vi "Set Controls Enable or Disable State Data Recorder.vi"(8 "error in (no error)":errorcluster, 10 "Refnum State":T2=enum."Start Live", 11 "Refnums In":T1) -> (0 "error out":errorcluster)   [LabVIEW 2017]
uses:
  Controls/Enabled State Control.ctl
  Controls/Refnums.ctl
  Controls/Recording Settings.ctl
  Controls/Operator Settings.ctl
  Controls/Operator.ctl
  Controls/Patient Settings.ctl
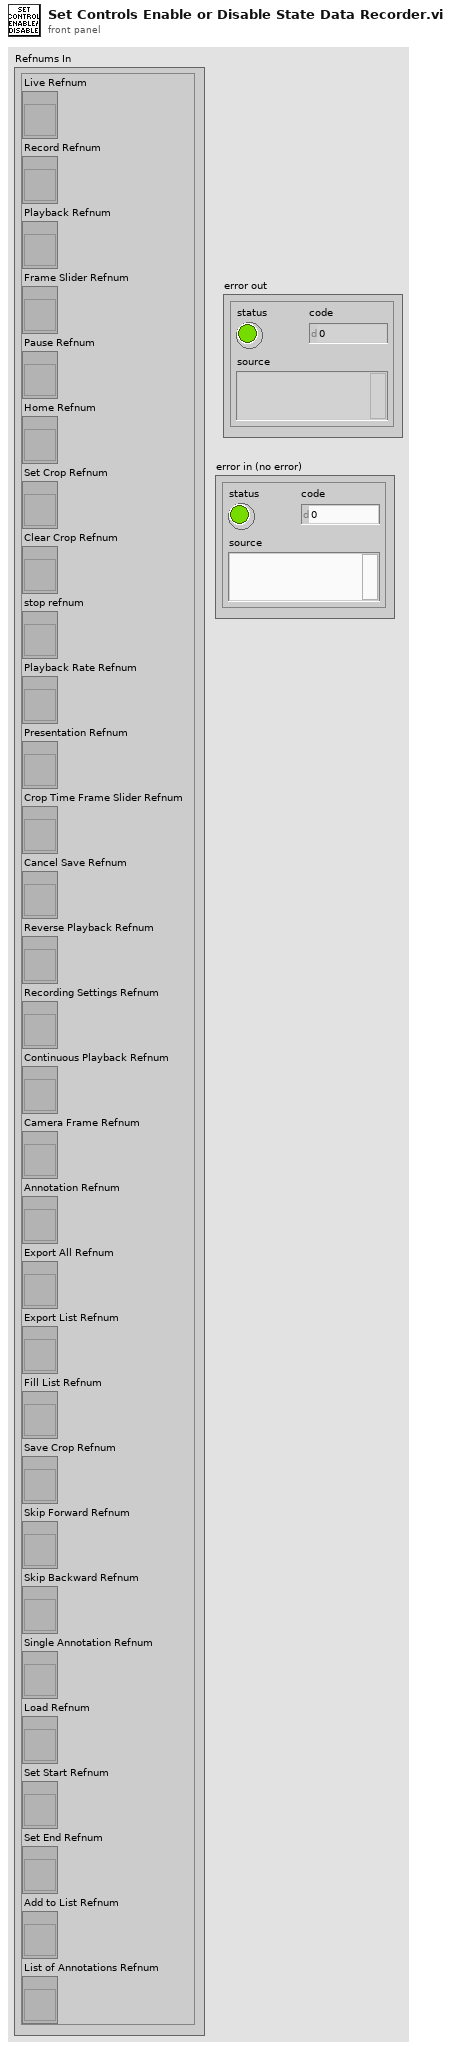
[diagram p1: front panel]
types:
  T1 = typedef "Refnums.ctl" = cluster{"Live Refnum":refnum<vi>, "Record Refnum":refnum<vi>, "Playback Refnum":refnum<vi>, "Frame Slider Refnum":refnum<vi>, "Pause Refnum":refnum<vi>, "Home Refnum":refnum<vi>, "Set Crop Refnum":refnum<vi>, "Clear Crop Refnum":refnum<vi>, "stop refnum":refnum<vi>, "Playback Rate Refnum":refnum<vi>, "Presentation Refnum":refnum<vi>, "Crop Time Frame Slider Refnum":refnum<vi>, "Cancel Save Refnum":refnum<vi>, "Reverse Playback Refnum":refnum<vi>, "Recording Settings Refnum":refnum<vi>, "Continuous Playback Refnum":refnum<vi>, "Camera Frame Refnum":refnum<vi>, "Annotation Refnum":refnum<vi>, "Export All Refnum":refnum<vi>, "Export List Refnum":refnum<vi>, "Fill List Refnum":refnum<vi>, "Save Crop Refnum":refnum<vi>, "Skip Forward Refnum":refnum<vi>, "Skip Backward Refnum":refnum<vi>, "Single Annotation Refnum":refnum<vi>, "Load Refnum":refnum<vi>, "Set Start Refnum":refnum<vi>, "Set End Refnum":refnum<vi>, "Add to List Refnum":refnum<vi>, "List of Annotations Refnum":refnum<vi>}
  T2 = typedef "Enabled State Control.ctl" = enum16{"Wait", "Start Live", "Start Recording", "Start Playback", "Shutdown"}
  T3 = enum8{"Enabled", "Disabled", "Disabled and Grayed Out"}
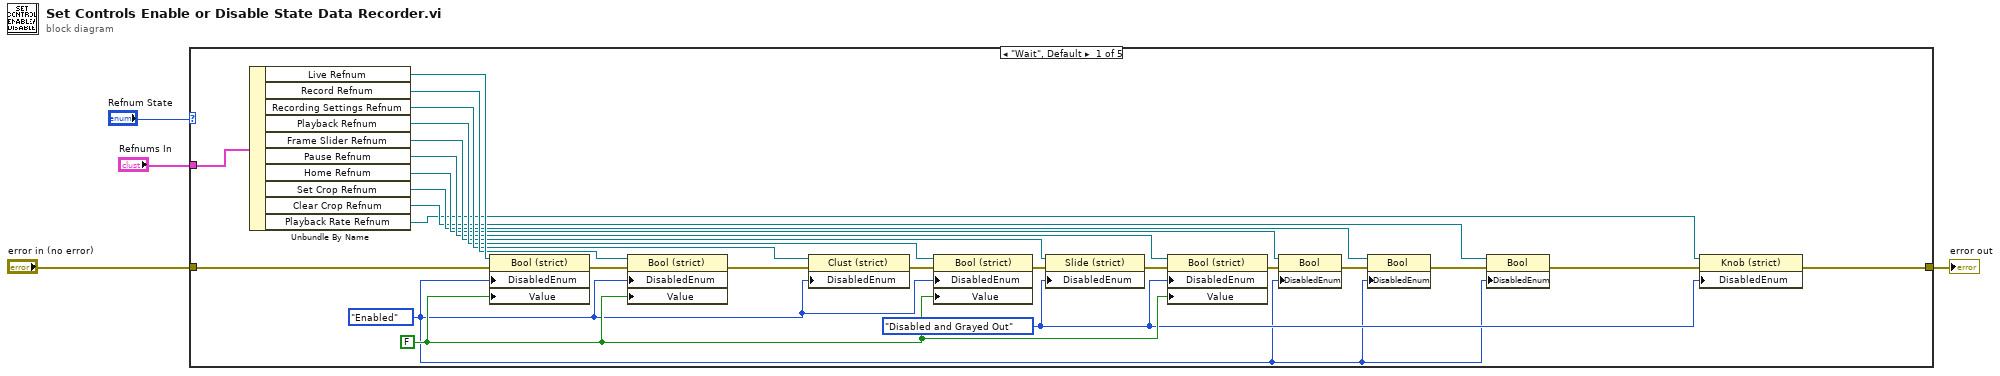
[diagram p0: block diagram]
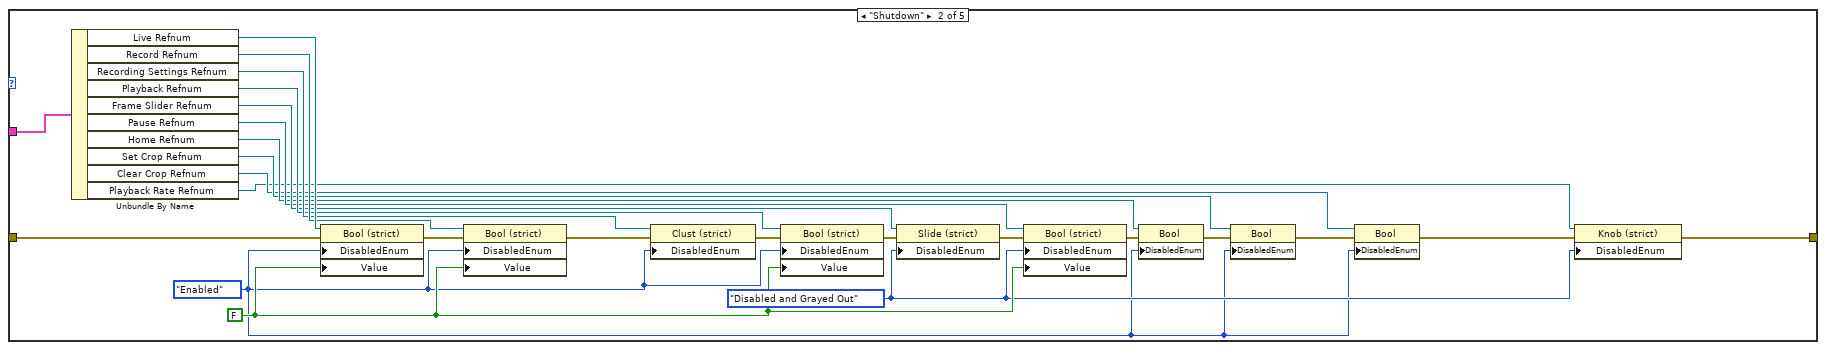
[diagram p2: hidden frame]
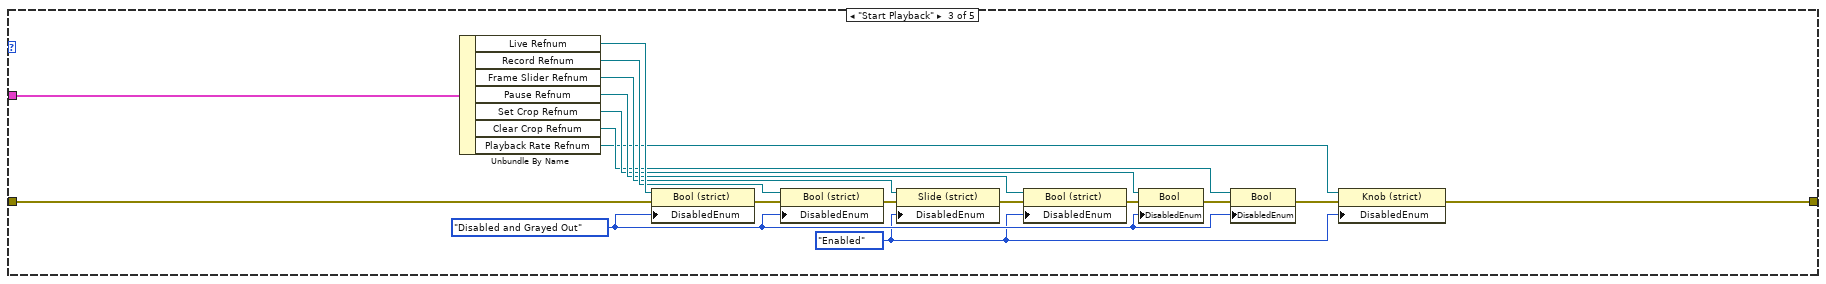
[diagram p3: hidden frame]
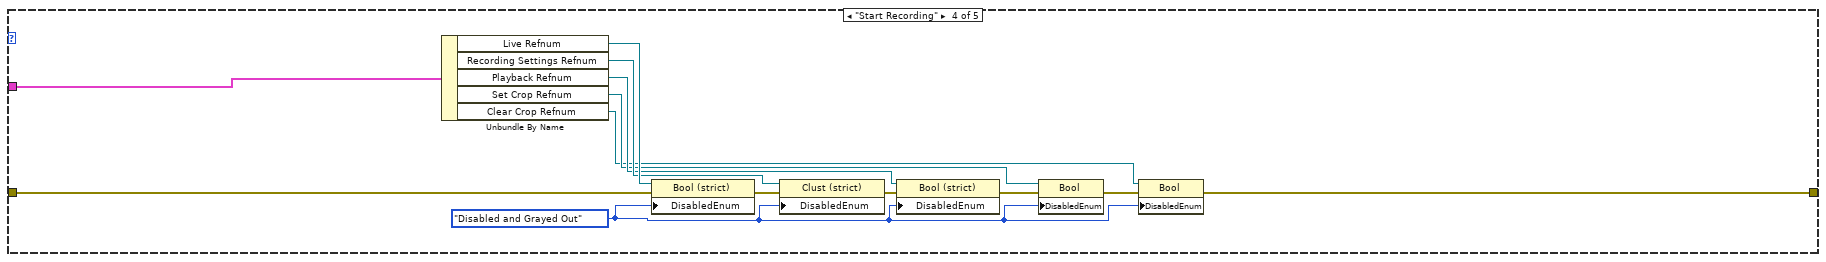
[diagram p4: hidden frame]
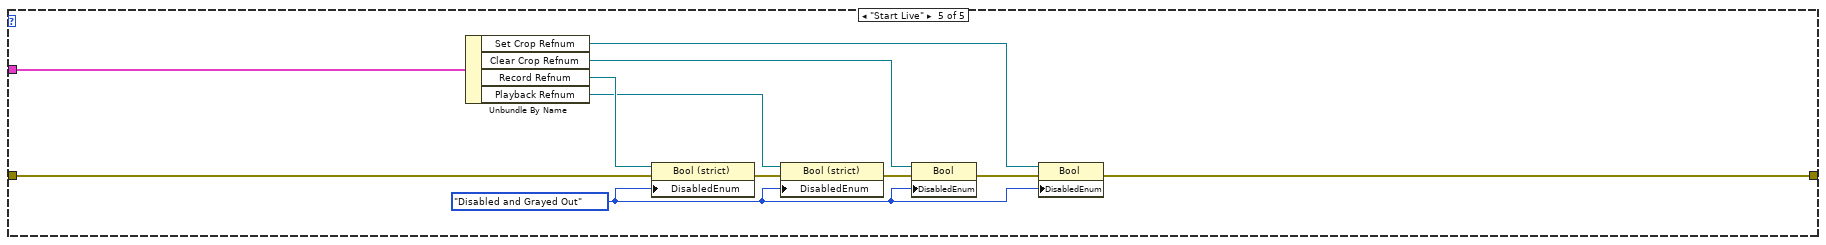
[diagram p5: hidden frame]
diagram:
  n1 = case shown="\"Wait\", Default" "Refnum State" {
    tunnel: "Refnums In" -> [w29 w54 w72 w85 w96]
    tunnel: "error in (no error)" -> [w19 w44 w65 w79 w92]
    tunnel: [w5 w30 w57 w74 w87] -> w4
    frame "Wait", Default {
      w9 = FALSE
      w7 = T3."Disabled and Grayed Out" ("Disabled")
      w6 = T3."Enabled" ("Disabled")
      n2 = Unbundle By Name(w29) -> ("Live Refnum"=w28:refnum<vi>, "Record Refnum"=w27:refnum<vi>, "Recording Settings Refnum"=w26:refnum<vi>, "Playback Refnum"=w25:refnum<vi>, "Frame Slider Refnum"=w24:refnum<vi>, "Pause Refnum"=w23:refnum<vi>, "Home Refnum"=w22:refnum<vi>, "Set Crop Refnum"=w21:refnum<vi>, "Clear Crop Refnum"=w20:refnum<vi>, "Playback Rate Refnum"=w8:refnum<vi>)
      n3 = property class="Bool (strict)"(reference=w28, error in=w19, "DisabledEnum"=w6, "Value"=w9) -> (error out=w18:errorcluster)  [unwired: 1 out]
      n4 = property class="Bool (strict)"(reference=w27, error in=w18, "DisabledEnum"=w6, "Value"=w9) -> (error out=w17:errorcluster)  [unwired: 1 out]
      n5 = property class="Clust (strict)"(reference=w26, error in=w17, "DisabledEnum"=w6) -> (error out=w16:errorcluster)  [unwired: 1 out]
      n6 = property class="Bool (strict)"(reference=w25, error in=w16, "DisabledEnum"=w6, "Value"=w9) -> (error out=w15:errorcluster)  [unwired: 1 out]
      n7 = property class="Slide (strict)"(reference=w24, error in=w15, "DisabledEnum"=w7) -> (error out=w14:errorcluster)  [unwired: 1 out]
      n8 = property class="Bool (strict)"(reference=w23, error in=w14, "DisabledEnum"=w7, "Value"=w9) -> (error out=w13:errorcluster)  [unwired: 1 out]
      n9 = property class="Bool"(reference=w22, error in=w13, "DisabledEnum"=w6) -> (error out=w12:errorcluster)  [unwired: 1 out]
      n10 = property class="Bool"(reference=w21, error in=w12, "DisabledEnum"=w6) -> (error out=w11:errorcluster)  [unwired: 1 out]
      n11 = property class="Bool"(reference=w20, error in=w11, "DisabledEnum"=w6) -> (error out=w10:errorcluster)  [unwired: 1 out]
      n12 = property class="Knob (strict)"(reference=w8, error in=w10, "DisabledEnum"=w7) -> (error out=w5:errorcluster)  [unwired: 1 out]
    }
    frame "Shutdown" {
      w34 = FALSE
      w32 = T3."Disabled and Grayed Out" ("Disabled")
      w31 = T3."Enabled" ("Disabled")
      n13 = Unbundle By Name(w54) -> ("Live Refnum"=w53:refnum<vi>, "Record Refnum"=w52:refnum<vi>, "Recording Settings Refnum"=w51:refnum<vi>, "Playback Refnum"=w50:refnum<vi>, "Frame Slider Refnum"=w49:refnum<vi>, "Pause Refnum"=w48:refnum<vi>, "Home Refnum"=w47:refnum<vi>, "Set Crop Refnum"=w46:refnum<vi>, "Clear Crop Refnum"=w45:refnum<vi>, "Playback Rate Refnum"=w33:refnum<vi>)
      n14 = property class="Bool (strict)"(reference=w53, error in=w44, "DisabledEnum"=w31, "Value"=w34) -> (error out=w43:errorcluster)  [unwired: 1 out]
      n15 = property class="Bool (strict)"(reference=w52, error in=w43, "DisabledEnum"=w31, "Value"=w34) -> (error out=w42:errorcluster)  [unwired: 1 out]
      n16 = property class="Clust (strict)"(reference=w51, error in=w42, "DisabledEnum"=w31) -> (error out=w41:errorcluster)  [unwired: 1 out]
      n17 = property class="Bool (strict)"(reference=w50, error in=w41, "DisabledEnum"=w31, "Value"=w34) -> (error out=w40:errorcluster)  [unwired: 1 out]
      n18 = property class="Slide (strict)"(reference=w49, error in=w40, "DisabledEnum"=w32) -> (error out=w39:errorcluster)  [unwired: 1 out]
      n19 = property class="Bool (strict)"(reference=w48, error in=w39, "DisabledEnum"=w32, "Value"=w34) -> (error out=w38:errorcluster)  [unwired: 1 out]
      n20 = property class="Bool"(reference=w47, error in=w38, "DisabledEnum"=w31) -> (error out=w37:errorcluster)  [unwired: 1 out]
      n21 = property class="Bool"(reference=w46, error in=w37, "DisabledEnum"=w31) -> (error out=w36:errorcluster)  [unwired: 1 out]
      n22 = property class="Bool"(reference=w45, error in=w36, "DisabledEnum"=w31) -> (error out=w35:errorcluster)  [unwired: 1 out]
      n23 = property class="Knob (strict)"(reference=w33, error in=w35, "DisabledEnum"=w32) -> (error out=w30:errorcluster)  [unwired: 1 out]
    }
    frame "Start Playback" {
      w61 = T3."Disabled and Grayed Out" ("Disabled")
      w56 = T3."Enabled" ("Disabled")
      n24 = Unbundle By Name(w72) -> ("Live Refnum"=w71:refnum<vi>, "Record Refnum"=w70:refnum<vi>, "Frame Slider Refnum"=w69:refnum<vi>, "Pause Refnum"=w68:refnum<vi>, "Set Crop Refnum"=w67:refnum<vi>, "Clear Crop Refnum"=w66:refnum<vi>, "Playback Rate Refnum"=w59:refnum<vi>)
      n25 = property class="Bool (strict)"(reference=w71, error in=w65, "DisabledEnum"=w61) -> (error out=w64:errorcluster)  [unwired: 1 out]
      n26 = property class="Bool (strict)"(reference=w70, error in=w64, "DisabledEnum"=w61) -> (error out=w60:errorcluster)  [unwired: 1 out]
      n27 = property class="Slide (strict)"(reference=w69, error in=w60, "DisabledEnum"=w56) -> (error out=w63:errorcluster)  [unwired: 1 out]
      n28 = property class="Bool (strict)"(reference=w68, error in=w63, "DisabledEnum"=w56) -> (error out=w55:errorcluster)  [unwired: 1 out]
      n29 = property class="Bool"(reference=w67, error in=w55, "DisabledEnum"=w61) -> (error out=w62:errorcluster)  [unwired: 1 out]
      n30 = property class="Bool"(reference=w66, error in=w62, "DisabledEnum"=w61) -> (error out=w58:errorcluster)  [unwired: 1 out]
      n31 = property class="Knob (strict)"(reference=w59, error in=w58, "DisabledEnum"=w56) -> (error out=w57:errorcluster)  [unwired: 1 out]
    }
    frame "Start Recording" {
      w75 = T3."Disabled and Grayed Out" ("Disabled")
      n32 = Unbundle By Name(w85) -> ("Live Refnum"=w84:refnum<vi>, "Recording Settings Refnum"=w83:refnum<vi>, "Playback Refnum"=w82:refnum<vi>, "Set Crop Refnum"=w81:refnum<vi>, "Clear Crop Refnum"=w80:refnum<vi>)
      n33 = property class="Bool (strict)"(reference=w84, error in=w79, "DisabledEnum"=w75) -> (error out=w76:errorcluster)  [unwired: 1 out]
      n34 = property class="Clust (strict)"(reference=w83, error in=w76, "DisabledEnum"=w75) -> (error out=w78:errorcluster)  [unwired: 1 out]
      n35 = property class="Bool (strict)"(reference=w82, error in=w78, "DisabledEnum"=w75) -> (error out=w73:errorcluster)  [unwired: 1 out]
      n36 = property class="Bool"(reference=w81, error in=w73, "DisabledEnum"=w75) -> (error out=w77:errorcluster)  [unwired: 1 out]
      n37 = property class="Bool"(reference=w80, error in=w77, "DisabledEnum"=w75) -> (error out=w74:errorcluster)  [unwired: 1 out]
    }
    frame "Start Live" {
      w86 = T3."Disabled and Grayed Out" ("Disabled")
      n38 = Unbundle By Name(w96) -> ("Set Crop Refnum"=w91:refnum<vi>, "Clear Crop Refnum"=w90:refnum<vi>, "Record Refnum"=w95:refnum<vi>, "Playback Refnum"=w94:refnum<vi>)
      n39 = property class="Bool (strict)"(reference=w95, error in=w92, "DisabledEnum"=w86) -> (error out=w93:errorcluster)  [unwired: 1 out]
      n40 = property class="Bool (strict)"(reference=w94, error in=w93, "DisabledEnum"=w86) -> (error out=w89:errorcluster)  [unwired: 1 out]
      n41 = property class="Bool"(reference=w90, error in=w89, "DisabledEnum"=w86) -> (error out=w88:errorcluster)  [unwired: 1 out]
      n42 = property class="Bool"(reference=w91, error in=w88, "DisabledEnum"=w86) -> (error out=w87:errorcluster)  [unwired: 1 out]
    }
  }
  "error out" <- w4
